vi "SIM Registry Update Continuous ICs.vi"(6 "Block Tag":string, 9 "IC limited":bool, 10 "IC":dbl, 11 "State data in":T1) -> (3 "State data out":T1)   [LabVIEW 2020]
uses:
  <vilib>/Simulation/Implementation/Shared/SIM solver state data.ctl
  <vilib>/Simulation/Implementation/Shared/SIM limit type.ctl
  <vilib>/Simulation/Implementation/Shared/SIM trigger type.ctl
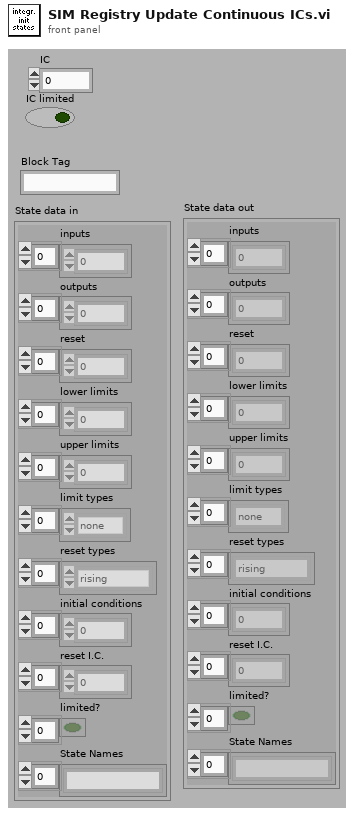
[diagram p1: front panel]
types:
  T1 = typedef "SIM solver state data.ctl" = cluster{"inputs":dbl[], "outputs":dbl[], "reset":dbl[], "lower limits":dbl[], "upper limits":dbl[], "limit types":T2[], "reset types":T3[], "initial conditions":dbl[], "reset I.C.":dbl[], "limited?":bool[], "State Names":string[]}
  T2 = typedef "SIM limit type.ctl" = enum16{"upper", "lower", "both", "none"}
  T3 = typedef "SIM trigger type.ctl" = enum16{"rising", "falling", "either", "none"}
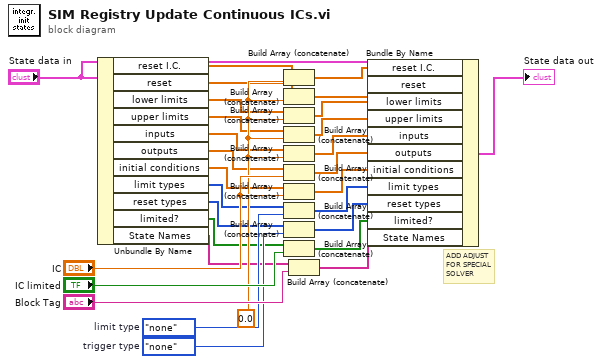
[diagram p0: block diagram]
diagram:
  w27 = SIM_trigger_type."none"  # trigger type
  w26 = SIM_limit_type."none"  # limit type
  w25 = 0.0 ("limited signal")
  # "ADD ADJUST\nFOR SPECIAL\nSOLVER"
  n1 = Unbundle By Name("State data in") -> ("reset I.C."=w1:dbl[], "reset"=w4:dbl[], "lower limits"=w6:dbl[], "upper limits"=w7:dbl[], "inputs"=w9:dbl[], "outputs"=w13:dbl[], "initial conditions"=w23:dbl[], "limit types"=w15:T2[], "reset types"=w17:T3[], "limited?"=w18:bool[], "State Names"=w19:string[])
  n2 = Build Array (concatenate)(w1, w25) -> (w3:dbl[])
  n3 = Build Array (concatenate)(w4, w25) -> (w5:dbl[])
  n4 = Build Array (concatenate)(w6, w25) -> (w8:dbl[])
  n5 = Build Array (concatenate)(w7, w25) -> (w11:dbl[])
  n6 = Build Array (concatenate)(w9, w25) -> (w10:dbl[])
  n7 = Build Array (concatenate)(w13, "IC") -> (w12:dbl[])
  n8 = Build Array (concatenate)(w23, "IC") -> (w14:dbl[])
  n9 = Build Array (concatenate)(w15, w26) -> (w16:T2[])
  n10 = Build Array (concatenate)(w17, w27) -> (w20:T3[])
  n11 = Build Array (concatenate)(w18, "IC limited") -> (w21:bool[])
  n12 = Build Array (concatenate)(w19, "Block Tag") -> (w22:string[])
  n13 = Bundle By Name(cluster="State data in", "reset I.C."=w3, "reset"=w5, "lower limits"=w8, "upper limits"=w11, "inputs"=w10, "outputs"=w12, "initial conditions"=w14, "limit types"=w16, "reset types"=w20, "limited?"=w21, "State Names"=w22) -> (→"State data out":T1)
